vi "Get Module Information.vi"(8 "error in":errorcluster, 11 "Module reference":refnum<k21>) -> (0 "error out":errorcluster, 2 "Module Information":T1 {"Module Code" format="%.0x"})   [LabVIEW 2015, in "SMI.lvlib" / "Module Detection.lvclass"]
uses:
  Module Detection.lvclass
  Controls/ModuleInformation.ctl
  <resource>/objmgr/cRIO.rc
  <resource>/objmgr/ni.var.rc
  <vilib>/regexp/Match Regular Expression.xnode
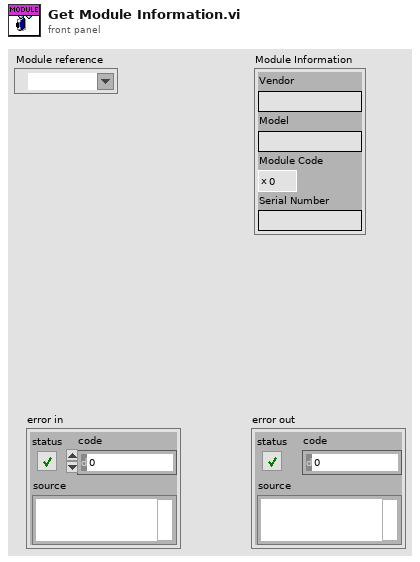
[diagram p1: front panel]
types:
  T1 = typedef "SMI.lvlib/Module Detection.lvclass/ModuleInformation.ctl" = cluster{"Vendor":string, "Model":string, "Module Code":u32, "Serial Number":string}
  T2 = cluster{"Slot":string, "Model":string, "VendorURL":string, "Channels":string, "Readable":string, "Writable":string, "ModbusAddress":string, "ChannelName":string, "ChannelRange":string, "TimeStamp":string, "ChannelType":string}
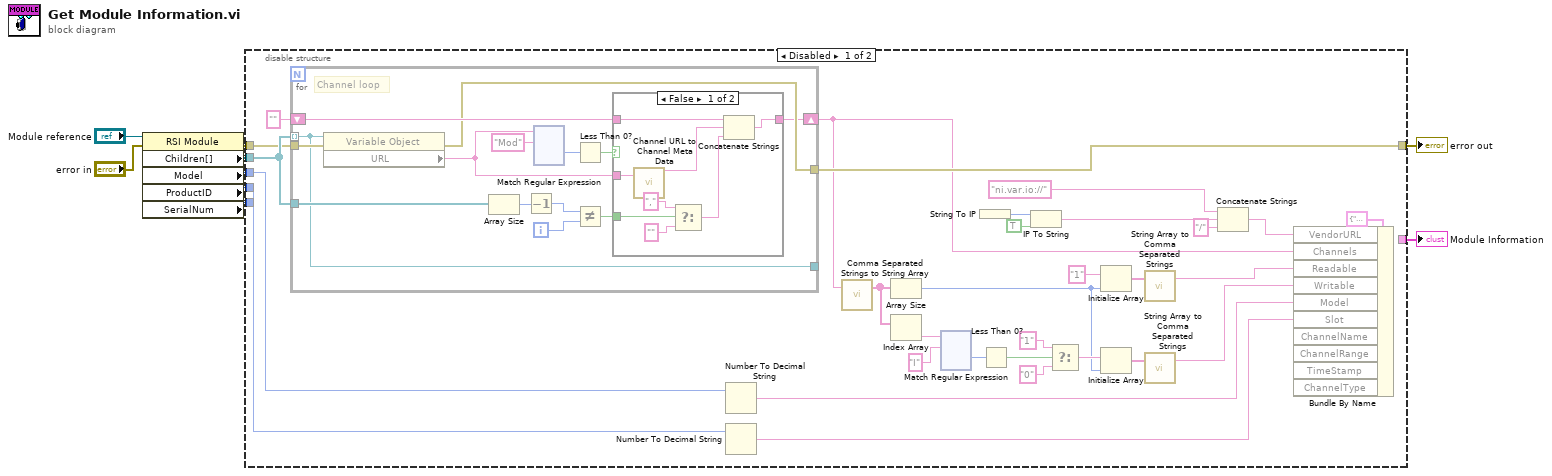
[diagram p0: block diagram]
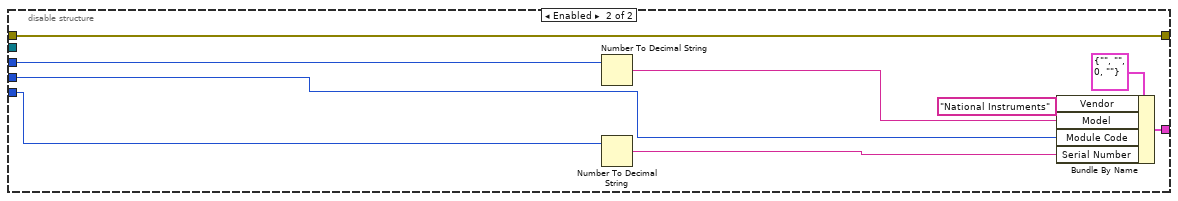
[diagram p3: hidden frame]
diagram:
  n1 = property class="RSI Module"(reference="Module reference", error in="error in") -> (error out=w6:errorcluster, "Children[]"=w9:refnum<k21>[], "Model"=w2:u32, "ProductID"=w3:u32, "SerialNum"=w1:u32)  [unwired: 1 out]
  n2 = disable-structure shown="Disabled" {
    disable-tunnel: w9 -> [w39 _]
    disable-tunnel: [_ w293] -> w7
    disable-tunnel: w6 -> [w37 w287]
    disable-tunnel: [w36 w287] -> w5
    disable-tunnel: w3 -> [w34 w286]
    disable-tunnel: w2 -> [w33 w292]
    disable-tunnel: w1 -> [_ w289]
    frame Disabled {
      n3 = for {
        tunnel: w39 -> [w151] mode=indexing
        tunnel: w39 -> [w161]
        shift-right: [w153] -> w29
        shift-left: "" -> [w156]
        tunnel: w37 -> [w155]
        tunnel: [w154] -> w36
        tunnel: [w151] -> _
        i -> [w158]
        # "Channel loop"
        n4 = property class="Variable Object"(reference=w151, error in=w155) -> (error out=w154:errorcluster, "URL"=w152:string)  [unwired: 1 out]
        n5 = Array Size(array=w161) -> (size(s)=w160:i32)
        n6 = Decrement(x=w160) -> (x-1=w159:i32)
        n7 = xnode "Match Regular Expression"("input string"=w152, "regular expression"="Mod") -> ("offset past match"=w163:i32)  [unwired: 4 in, 4 out]
        n8 = Less Than 0?(x=w163) -> (x < 0?=w162:bool)
        n9 = Not Equal?(x=w159, y=w158) -> (x != y?=w157:bool)
        n10 = case shown="False" w162 {
          tunnel: w152 -> [w172 _]
          tunnel: w157 -> [w170 _]
          tunnel: [w166 w173] -> w153
          tunnel: w156 -> [w165 w173]
          frame False {
            n11 = call "Channel URL to Channel Meta Data.vi"("Channel URL"=w172) -> ("Channel Name"=w171:string)  [unwired: 16 in, 2 out]
            n12 = Select(t=",", s=w170, f="") -> (s? t:f=w168:string)
            n13 = Concatenate Strings(w165, w171, w168) -> (w166:string)
          }
          frame True {
          }
        }
      }
      n14 = Number To Decimal String(number=w33) -> (decimal integer string=w30:string)  [unwired: 1 in]
      n15 = Number To Decimal String(number=w34) -> (decimal integer string=w35:string)  [unwired: 1 in]
      n16 = call "Comma Separated Strings to String Array.vi"("Comma Separated Strings"=w29) -> ("String Array"=w12:string[])  [unwired: 18 in]
      n17 = Array Size(array=w12) -> (size(s)=w15:i32)
      n18 = Index Array(array=w12) -> (element=w11:string)  [unwired: 1 in]
      n19 = xnode "Match Regular Expression"("input string"=w11, "regular expression"="I") -> ("offset past match"=w21:i32)  [unwired: 4 in, 4 out]
      n20 = String To IP() -> (0:w28:u32)  [unwired: 1 in]
      n21 = Less Than 0?(x=w21) -> (x < 0?=w20:bool)
      n22 = IP To String(1:TRUE ("dot notation? (F)"), 2:w28) -> (0:w26:string)
      n23 = Select(t="1" ("regular expression"), s=w20, f="0" ("regular expression")) -> (s? t:f=w17:string)
      n24 = Initialize Array("1" ("element"), w15) -> (w13:string[])
      n25 = Initialize Array(w17, w15) -> (w16:string[])
      n26 = call "String Array to Comma Separated Strings.vi"("String Array"=w13) -> ("Comma Separated Strings"=w32:string)  [unwired: 18 in]
      n27 = call "String Array to Comma Separated Strings.vi"("String Array"=w16) -> ("Comma Separated Strings"=w31:string)  [unwired: 18 in]
      n28 = Concatenate Strings("ni.var.io://", w26, "/" ("string")) -> (w23:string)
      n29 = Bundle By Name(cluster=T2 {"Slot"="", "Model"="", "VendorURL"="", "Channels"="", "Readable"="", "Writable"="", "ModbusAddress"="", "ChannelName"="", "ChannelRange"="", "TimeStamp"="", "ChannelType"=""} ("Channel info"), "VendorURL"=w23, "Channels"=w29, "Readable"=w32, "Writable"=w31, "Model"=w30, "Slot"=w35) -> ()  [unwired: 4 in, 1 out]
    }
    frame Enabled {
      n30 = Number To Decimal String(number=w292) -> (decimal integer string=w290:string)  [unwired: 1 in]
      n31 = Number To Decimal String(number=w289) -> (decimal integer string=w288:string)  [unwired: 1 in]
      n32 = Bundle By Name(cluster=T1 {"Vendor"="", "Model"="", "Module Code"=0, "Serial Number"=""} ("Channel info"), "Vendor"="National Instruments", "Model"=w290, "Module Code"=w286, "Serial Number"=w288) -> (w293:T1)
    }
  }
  "error out" <- w5
  "Module Information" <- w7
